vi "Remove Array from Hash Table.vi"(8 "error in (no error)":errorcluster caption="错误输入（无错误）", 11 "Contstant Base 输入":refnum<class "Tag Data.lvclass"> caption="DNL_LabVIEW Object in") -> (0 "error out":errorcluster caption="错误输出", 3 "Contstant Base 输出":refnum<class "Tag Data.lvclass"> caption="DNL_LabVIEW Object out")   [LabVIEW 2013, in "Tag Data.lvclass"]
uses:
  Tag Data.lvclass
panel:
  in  "Name":string[](array[string])
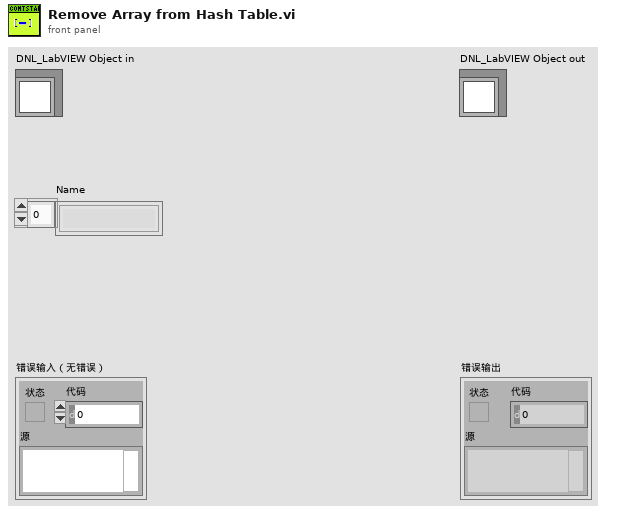
[diagram p1: front panel]
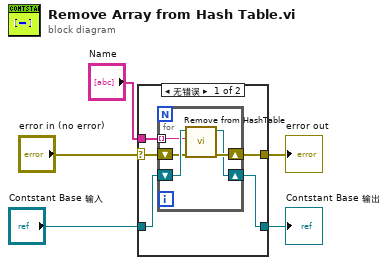
[diagram p0: block diagram]
diagram:
  n1 = case shown="无错误" "error in (no error)" {
    selector: "error in (no error)" -> [w8 w17]
    tunnel: [w7 w17] -> w4
    tunnel: [w6 w16] -> w2
    tunnel: "Contstant Base 输入" -> [w10 w16]
    tunnel: "Name" -> [w9 _]
    frame No Error {
      n2 = for {
        shift-right: [w11] -> w6
        shift-left: w10 -> [w15]
        tunnel: w9 -> [w14] mode=indexing
        shift-right: [w12] -> w7
        shift-left: w8 -> [w13]
        n3 = call-dynamic "Remove from HashTable.vi"("error in (no error)"=w13, "Name"=w14, "Contstant Base 输入"=w15) -> ("error out"=w12:errorcluster, "Contstant Base 输出"=w11:refnum<class "Tag Data.lvclass">)  [unwired: 7 in]
      }
    }
    frame Error {
    }
  }
  "error out" <- w4
  "Contstant Base 输出" <- w2
